vi "DDS Read RAM register.vi"(6 "channel number (1)":u8=1 min=1 max=4 step=1, 8 "error in (no error)":errorcluster, 9 "# of Words":u16, 10 "Register":T3=enum."RAM", 11 "DDS ref in":T1={"NI USB-8451 device reference"="", "DIO port"=0, "Serial Clock Rate [kHz]"=1000}) -> (0 "error out":errorcluster, 2 "RAM data":u8[][](array[numeric]), 3 "DDS ref out":T1={"NI USB-8451 device reference"="", "DIO port"=0, "Serial Clock Rate [kHz]"=1000})   [LabVIEW 2013]
doc: "Read the RAM and Profile settings to check that the DDS board was programmed correctly."
uses:
  AD9910 registers.ctl
  DDS_box_device_reference.ctl
  <vilib>/ni845x/ni845x.llb/ni845xControl.ctl
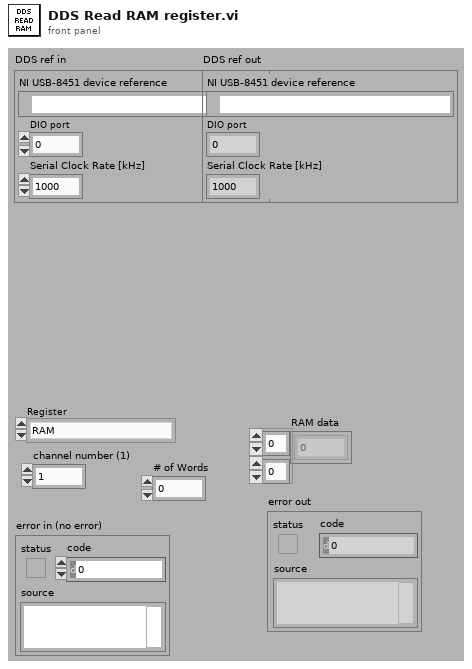
[diagram p1: front panel]
types:
  T1 = typedef "DDS_box_device_reference.ctl" = cluster{"NI USB-8451 device reference":T2, "DIO port":u8, "Serial Clock Rate [kHz]":u16}
  T2 = typedef "ni845xControl.ctl" = refnum<k21>
  T3 = typedef "AD9910 registers.ctl" = enum16{"CFR1", "CFR2", "CFR3", "Auxiliary DAC Control", "I/0 Update Rate", "Frequency Tuning Word", "Phase Offset Word", "Amplitude Scale Factor", "Multichip Sync", "Digital Ramp Limit", "Digital Ramp Step Size", "Digital Ramp Rate", "Single Tone Profile 0", "Single Tone Profile 1", "Single Tone Profile 2", "Single Tone Profile 3", "Single Tone Profile 4", "Single Tone Profile 5", "Single Tone Profile 6", "Single Tone Profile 7", "RAM Profile 0", "RAM Profile 1", "RAM Profile 2", "RAM Profile 3", "RAM Profile 4", "RAM Profile 5", "RAM Profile 6", "RAM Profile 7", "RAM"}
  T4 = typedef "ni845xSpiScriptControl.ctl" = refnum<k20>
  T5 = typedef "DDS CS pins.ctl" = enum8{"IO reset", "Ch. 4 CS", "Ch. 3 CS", "Ch. 2 CS", "Ch. 1 CS"}
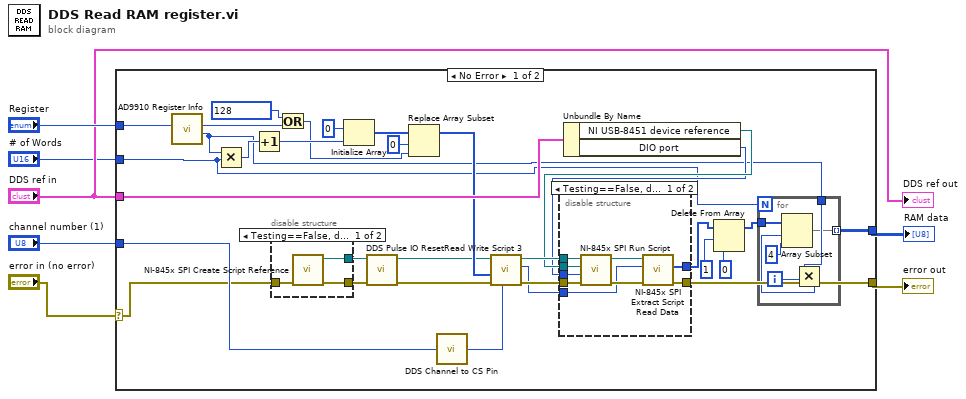
[diagram p0: block diagram]
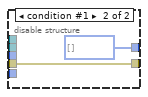
[diagram p2: hidden frame]
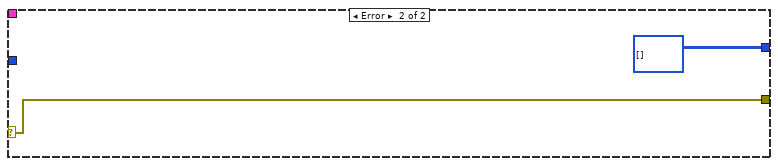
[diagram p4: hidden frame]
diagram:
  n1 = case shown="No Error" "error in (no error)" {
    selector: "error in (no error)" -> [w8 w60]
    tunnel: "DDS ref in" -> [w38 _]
    tunnel: "Register" -> [w35 _]
    tunnel: [w18 w60] -> w5
    tunnel: "channel number (1)" -> [w24 _]
    tunnel: "# of Words" -> [w9 _]
    tunnel: [w14 u8[][] []] -> w1
    frame No Error {
      n2 = call "AD9910 Register Info.vi"("Register"=w35) -> ("Number of Bytes"=w15:i32, "Address"=w27:u8)  [unwired: 9 in]
      n3 = Multiply(x=w15, y=w9) -> (x*y=w17:i32)
      n4 = Increment(x=w17) -> (x+1=w28:i32)
      n5 = disable-structure shown="Testing==False, default" {
        disable-tunnel: w8 -> [w58 w59]
        disable-tunnel: [w57 _] -> w37
        disable-tunnel: [w56 w59] -> w36
        frame condition #0 (active) {
          n6 = call <vilib>:"NI-845x SPI Create Script Reference.vi"("error in (no error)"=w58) -> ("error out"=w56:errorcluster, "spi script reference"=w57:T4)  [unwired: 9 in]
        }
        frame condition #1 {
        }
      }
      n7 = Or(x=u8 128, y=w27) -> (x .or. y?=w25:u8)
      n8 = Initialize Array(u8 0 ("element"), w28) -> (w33:u8[])
      n9 = call "DDS Pulse IO Reset.vi"("error in (no error)"=w36, "spi script reference in"=w37) -> ("error out"=w30:errorcluster, "spi script reference out"=w29:T4)  [unwired: 8 in]
      n10 = Replace Array Subset(array=w33, new element=w25, index=0) -> (w31:u8[])
      n11 = call "DDS Channel to CS Pin.vi"("channel number (1)"=w24) -> ("CS pin"=w23:T5)
      n12 = call "Read Write Script 3.vi"("chip select (0)"=w23, "error in (no error)"=w30, "Write Data"=w31, "spi script reference in"=w29) -> ("error out"=w22:errorcluster, "script read index"=w16:u32, "spi script reference out"=w21:T4)  [unwired: 5 in]
      n13 = Unbundle By Name(w38) -> ("NI USB-8451 device reference"=w20:T2, "DIO port"=w19:u8)
      n14 = disable-structure shown="Testing==False, default" {
        disable-tunnel: w22 -> [w53 w55]
        disable-tunnel: w21 -> [w52 _]
        disable-tunnel: w20 -> [w51 _]
        disable-tunnel: w19 -> [w50 _]
        disable-tunnel: [w47 w55] -> w18
        disable-tunnel: [w46 u8[] [] ("read data")] -> w12
        disable-tunnel: w16 -> [w45 _]
        frame condition #0 (active) {
          n15 = call <vilib>:"NI-845x SPI Run Script.vi"("error in (no error)"=w53, "port (0)"=w50, "device reference in"=w51, "spi script reference in"=w52) -> ("error out"=w49:errorcluster, "spi script reference out"=w48:T4)  [unwired: 5 in, 1 out]
          n16 = call <vilib>:"NI-845x SPI Extract Script Read Data.vi"("error in (no error)"=w49, "script read index"=w45, "spi script reference in"=w48) -> ("error out"=w47:errorcluster, "read data"=w46:u8[])  [unwired: 6 in, 1 out]
        }
        frame condition #1 {
        }
      }
      n17 = Delete From Array(array=w12, length=1, index=0) -> (array with subset deleted=w13:u8[])  [unwired: 1 out]
      n18 = for {
        N: w9 -> [_]
        tunnel: w13 -> [w44]
        tunnel: w15 -> [w42]
        tunnel: [w39] -> w14 mode=indexing
        i -> [w43]
        n19 = Multiply(x=w42, y=w43) -> (x*y=w41:i32)
        n20 = Array Subset(array=w44, index=w41, length=4) -> (w39:u8[])
      }
    }
    frame Error {
    }
  }
  "error out" <- w5
  "RAM data" <- w1
  "DDS ref out" <- "DDS ref in"
